vi "Count_Events.vi"(8 "error in (no error)":errorcluster, 11 "Constraints":T1) -> (0 "error out":errorcluster, 3 "Number of Matching Events":i32)   [LabVIEW 2011]
uses:
  Constraints.ctl
  <vilib>/addons/database/Auxilliary.llb/DB Tools Cursor Type.ctl
  <vilib>/addons/database/Connection.llb/Conn Execute.vi
  <vilib>/addons/database/Recordset.llb/Rec Fetch Recordset Data (R).vi
  <vilib>/addons/database/Recordset.llb/Rec Destroy - Connection.vi
  <vilib>/addons/database/_DB Variant To Data/Database Variant To Data.xnode
  <vilib>/addons/database/NI_Database_API.lvlib
panel:
  out "Names SQL Query Sintax":string
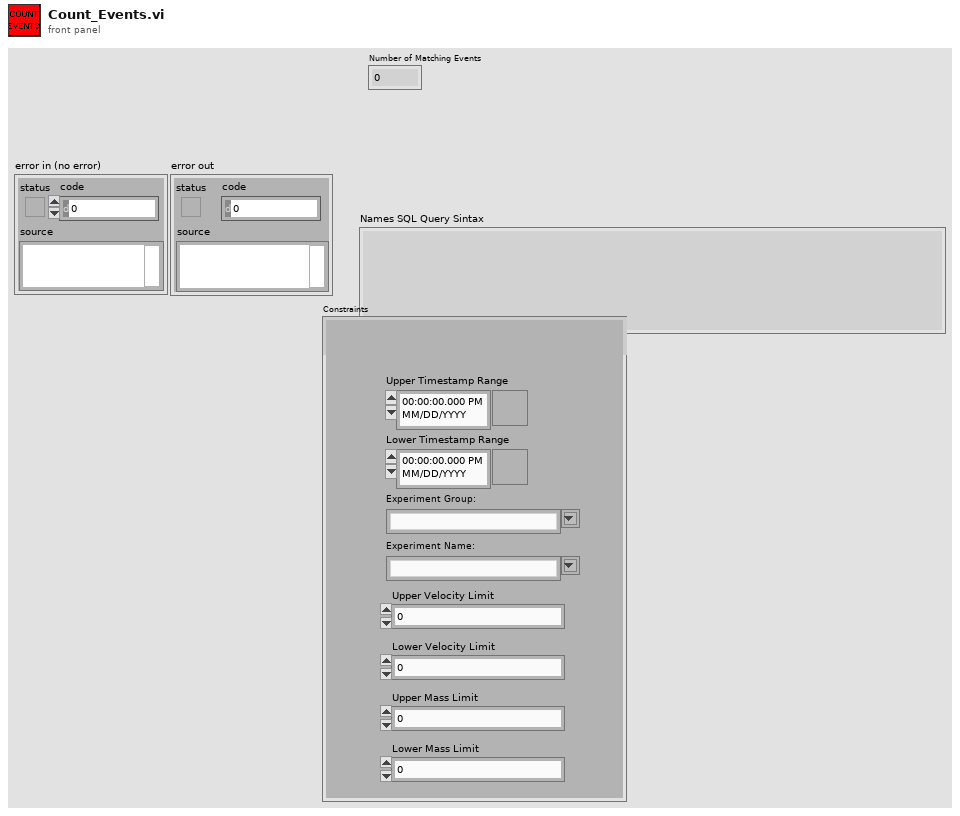
[diagram p1: front panel]
types:
  T1 = typedef "Constraints.ctl" = cluster{"Upper Timestamp Range":timestamp, "Lower Timestamp Range":timestamp, "Experiment Group:":string, "Experiment Name:":string, "Upper Velocity Limit":dbl, "Lower Velocity Limit":dbl, "Upper Mass Limit":dbl, "Lower Mass Limit":dbl}
  T2 = typedef "NI_Database_API.lvlib/DB Tools Cursor Type.ctl" = enum16{"forward-only", "keyset", "dynamic", "static"}
  T3 = typedef "NI_Database_API.lvlib/Conn ObjectReference.ctl" = refnum<k1>
  T4 = typedef "NI_Database_API.lvlib/Rec ObjectReference.ctl" = refnum<k1>
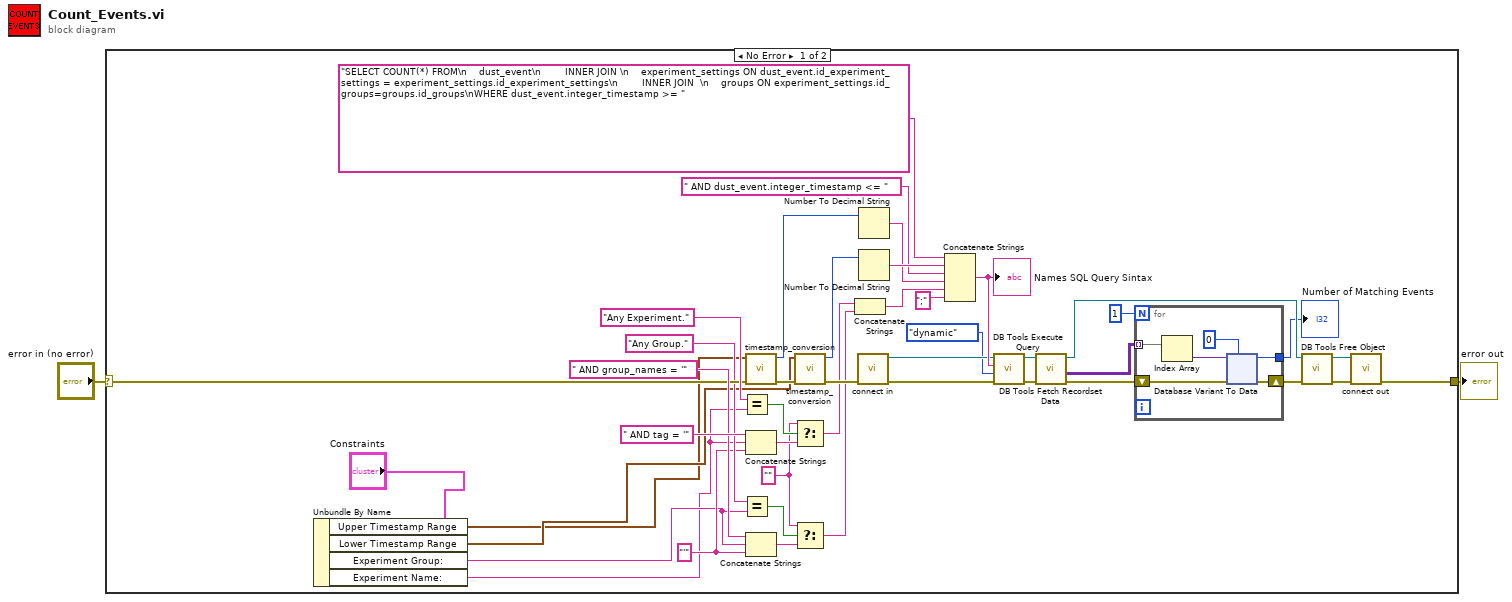
[diagram p0: block diagram]
diagram:
  n1 = case shown="No Error" "error in (no error)" {
    selector: "error in (no error)" -> [w21 w84]
    tunnel: [w18 w84] -> w1
    frame No Error {
      w15 = "'" ("string")
      w13 = "" ("t")
      n2 = Unbundle By Name("Constraints") -> ("Upper Timestamp Range"=w6:timestamp, "Lower Timestamp Range"=w7:timestamp, "Experiment Group:"=w4:string, "Experiment Name:"=w3:string)
      n3 = Equal?(x="Any Experiment.", y=w3) -> (x = y?=w32:bool)
      n4 = Equal?(x="Any Group.", y=w4) -> (x = y?=w31:bool)
      n5 = call "timestamp_conversion.vi"("error in (no error)"=w21, "Time Stamp"=w6) -> ("error out"=w23:errorcluster, "Integer Time"=w25:i64)  [unwired: 7 in]
      n6 = Concatenate Strings(" AND tag = '" ("string"), w3, w15) -> (w30:string)
      n7 = Concatenate Strings(" AND group_names = '" ("string"), w4, w15) -> (w29:string)
      n8 = call "timestamp_conversion.vi"("error in (no error)"=w23, "Time Stamp"=w7) -> ("error out"=w22:errorcluster, "Integer Time"=w24:i64)  [unwired: 7 in]
      n9 = Select(t=w13, s=w32, f=w30) -> (s? t:f=w14:string)
      n10 = Select(t=w13, s=w31, f=w29) -> (s? t:f=w5:string)
      n11 = Concatenate Strings(w14, w5) -> (w12:string)
      n12 = call "connect in.vi"("error in (no error)"=w22) -> ("error out"=w37:errorcluster, "Database Connection"=w38:T3)  [unwired: 6 in, 1 out]
      n13 = Number To Decimal String(number=w25) -> (decimal integer string=w19:string)  [unwired: 1 in]
      n14 = Number To Decimal String(number=w24) -> (decimal integer string=w35:string)  [unwired: 1 in]
      n15 = Concatenate Strings("SELECT COUNT(*) FROM\n    dust_event\n        INNER JOIN \n    experiment_settings ON dust_event.id_experiment_settings = experiment_settings.id_experiment_settings\n        INNER JOIN  \n    groups ON experiment_settings.id_groups=groups.id_groups\nWHERE dust_event.integer_timestamp >= " ("string"), w35, " AND dust_event.integer_timestamp <= " ("string"), w19, w12, ";" ("string")) -> (w43:string)
      "Names SQL Query Sintax" <- w43
      n16 = call-poly <vilib>:"DB Tools Execute Query.vi"("error in (no error)"=w37, "cursor type"=DB_Tools_Cursor_Type."dynamic", "SQL query"=w43, "connection reference"=w38) -> ("error out"=w44:errorcluster, "recordset reference"=w45:T4)  [unwired: 4 in]
      n17 = call-poly <vilib>:"DB Tools Fetch Recordset Data.vi"("error in (no error)"=w44, "recordset reference"=w45) -> ("error out"=w40:errorcluster, "recordset data"=w11:variant[][], "recordset reference out"=w42:T4)  [unwired: 3 in]
      n18 = for {
        N: 1 -> [_]
        tunnel: w11 -> [w51] mode=indexing
        shift-right: [w48] -> w39
        shift-left: w40 -> [w49]
        tunnel: [w46] -> w9
        n19 = Index Array(array=w51) -> (element=w50:variant)  [unwired: 1 in]
        n20 = xnode "Database Variant To Data"("database variant"=w50, "error in"=w49, "type"=0) -> ("data"=w46:i32, "error out"=w48:errorcluster)
      }
      "Number of Matching Events" <- w9
      n21 = call-poly <vilib>:"DB Tools Free Object.vi"("error in (no error)"=w39, "recordset reference"=w42) -> ("error out"=w41:errorcluster, "connection reference"=w36:T3)  [unwired: 8 in]
      n22 = call "connect out.vi"("error in (no error)"=w41, "connection reference"=w36) -> ("error out"=w18:errorcluster)  [unwired: 9 in]
    }
    frame Error {
    }
  }
  "error out" <- w1
